vi "Timeout.vi"(8 "error in (no error)":errorcluster, 10 "Data":variant, 11 "Vacuum in":refnum<class "Vacuum.lvclass">) -> (0 "error out":errorcluster, 3 "Vacuum out":refnum<class "Vacuum.lvclass">)   [LabVIEW 2015, in "AMS UI.lvlib" / "Vacuum.lvclass"]
uses:
  Vacuum.lvclass
  AMS Gas Actor/AMS Gas Actor.lvclass
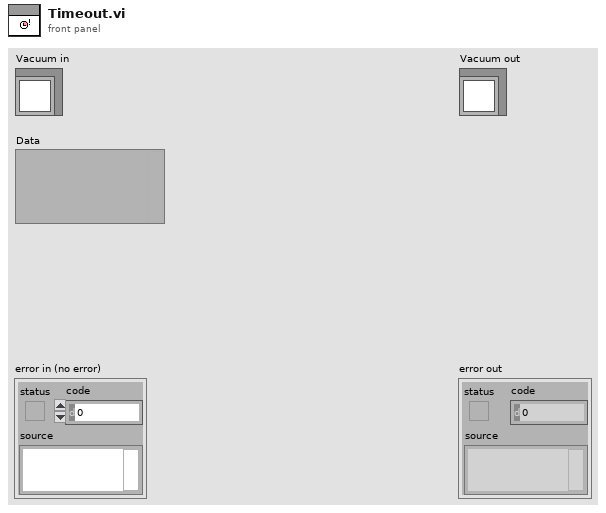
[diagram p1: front panel]
types:
  T1 = typedef "FP Control Refs Cluster.ctl" = cluster{"Liquid N Valve References":T2, "Main Line Valve Refs":T3, "Transfer Line Container":refnum<vi>, "Storage Containers":refnum<vi>[], "Sample Refs":T4, "Syringe Ctrl Refs ":T5, "Baratrons Chart":refnum<vi>, "Capillary Container":refnum<vi>, "Preparation Container":refnum<vi>, "Monkey Mode":refnum<vi>}
  T2 = typedef "Liquid N Valve Ref Cluster.ctl" = cluster{"Cold Bath H2O HV 100":refnum<vi>, "Cold Bath Cleaning HV 101":refnum<vi>, "Cold Bath Storage 1 HV 102":refnum<vi>, "Cold Bath Storage 2 HV 103":refnum<vi>, "Cold Bath Storage 3 HV 104":refnum<vi>, "Cold Bath Storage 4 HV 105":refnum<vi>, "Cold Bath Syringe HV 106":refnum<vi>, "Liquid N Master Valve HV 107":refnum<vi>}
  T3 = typedef "Main Line Valve Ref Cluster.ctl" = cluster{"Turbo Valve DV313":refnum<vi>, "Prep Line Valve 0 DV300":refnum<vi>, "Storage Valves":refnum<vi>[]}
  T4 = typedef "Sample Valve Refs.ctl" = cluster{"Valves":cluster{"Sample 5 DV318":refnum<vi>, "Sample 4 DV317":refnum<vi>, "Sample 3 DV316":refnum<vi>, "Sample 2 DV315":refnum<vi>, "Sample 1 DV314":refnum<vi>}, "Lines":cluster{"Sample 1":refnum<vi>, "Sample 2":refnum<vi>, "Sample 3":refnum<vi>, "Sample 4":refnum<vi>, "Sample 5":refnum<vi>}}
  T5 = typedef "Syringe Ctrl Refs.ctl" = cluster{"Syringe Home":refnum<vi>, "Syringe Freeze":refnum<vi>, "Syringe TC":refnum<vi>, "Syringe Container":refnum<vi>}
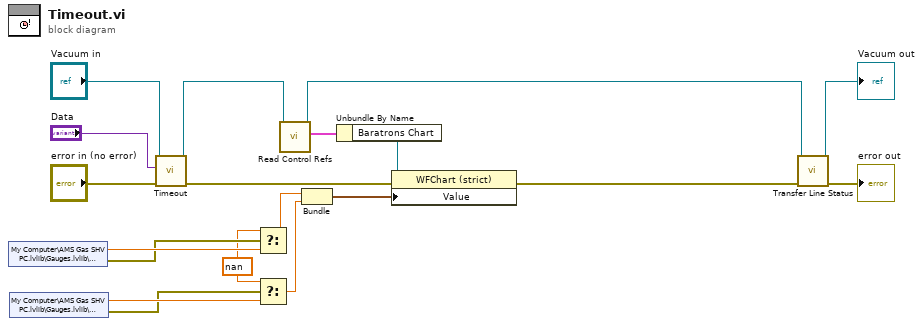
[diagram p0: block diagram]
diagram:
  w5 = nan ("t")
  n1 = shared-variable "My Computer\\AMS Gas SHV PC.lvlib\\Gauges.lvlib\\Baratron 1"() -> (w14:dbl, error out=w13:errorcluster)  [unwired: 1 in]
  n2 = shared-variable "My Computer\\AMS Gas SHV PC.lvlib\\Gauges.lvlib\\Baratron 2"() -> (w12:dbl, error out=w11:errorcluster)  [unwired: 1 in]
  n3 = call-parent "Timeout.vi"("error in (no error)"="error in (no error)", "Data"="Data", "eActor in"="Vacuum in") -> ("error out"=w18:errorcluster, "eActor out"=w4:refnum<class "Vacuum.lvclass">)  [unwired: 7 in]
  n4 = Select(t=w5, s=w13, f=w14) -> (s? t:f=w6:dbl)
  n5 = Select(t=w5, s=w11, f=w12) -> (s? t:f=w2:dbl)
  n6 = call-dynamic "Read Control Refs.vi"("AMS Gas Actor in"=w4) -> ("Control Refs"=w9:T1, "AMS Gas Actor out"=w3:refnum<class "Vacuum.lvclass">)  [unwired: 9 in]
  n7 = Bundle("Double"=w6, "Double"=w2) -> (w7:cluster{"Double":dbl, "Double":dbl})  [unwired: 1 in]
  n8 = Unbundle By Name(w9) -> ("Baratrons Chart"=w8:refnum<vi>)
  n9 = property class="WFChart (strict)"(reference=w8, error in=w18, "Value"=w7) -> (error out=w1:errorcluster)  [unwired: 1 out]
  n10 = call "Transfer Line Status.vi"("error in (no error)"=w1, "Vacuum in"=w3) -> ("error out"=→"error out":errorcluster, "Vacuum out"=→"Vacuum out":refnum<class "Vacuum.lvclass">)  [unwired: 8 in]
